vi "WPI_CameraGet Numeric Sensor Property.vi"(8 "error in (no error)":errorcluster, 10 "Property Name":string, 11 "CameraDevRef":T1) -> (0 "error out":errorcluster, 2 "Value":i32, 3 "CameraDevRef dup":T1)   [LabVIEW 2017]
doc: "This software is licensed. Open the labview\\readme\\WPI Robotics Library Open Source License.txt file for more information."
uses:
  <vilib>/Rock Robotics/WPI/Camera/WPI_CameraDevRef.ctl
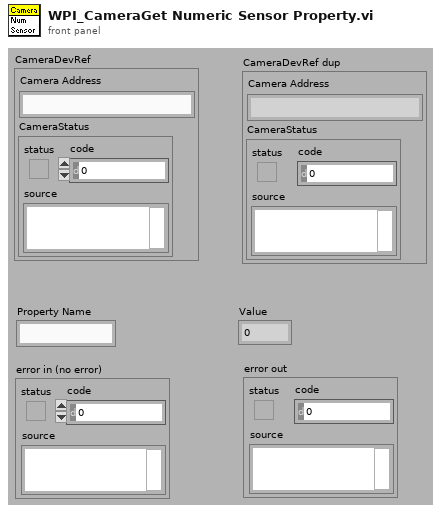
[diagram p1: front panel]
types:
  T1 = typedef "WPI_CameraDevRef.ctl" = cluster{"Camera Address":string, "CameraStatus":errorcluster}
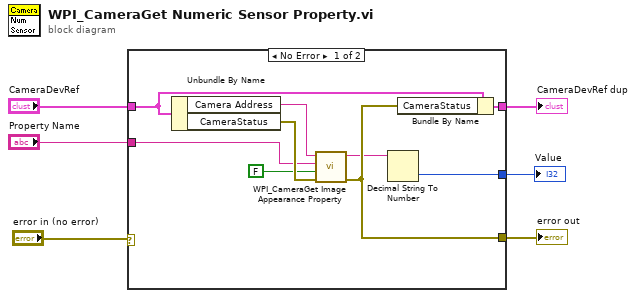
[diagram p0: block diagram]
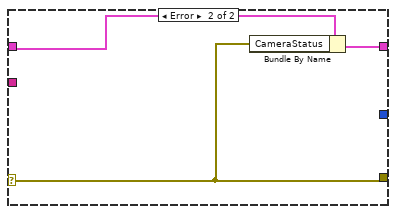
[diagram p2: hidden frame]
diagram:
  n1 = case shown="No Error" "error in (no error)" {
    selector: "error in (no error)" -> [_ w16]
    tunnel: "Property Name" -> [w10 _]
    tunnel: [w15 _] -> w5
    tunnel: [w11 w16] -> w4
    tunnel: "CameraDevRef" -> [w14 w17]
    tunnel: [w13 w18] -> w2
    frame No Error {
      n2 = Unbundle By Name(w14) -> ("Camera Address"=w9:string, "CameraStatus"=w12:errorcluster)
      n3 = call <vilib>:"WPI_CameraGet Image Appearance Property.vi"("error in (no error)"=w12, "Appearance"=FALSE, "Prop String"=w10, "address"=w9) -> ("error out"=w11:errorcluster, "Value"=w8:string)  [unwired: 6 in]
      n4 = Decimal String To Number(string=w8) -> (number=w15:i32)  [unwired: 3 out]
      n5 = Bundle By Name(cluster=w14, "CameraStatus"=w11) -> (w13:T1)
    }
    frame Error {
      n6 = Bundle By Name(cluster=w17, "CameraStatus"=w16) -> (w18:T1)
    }
  }
  "error out" <- w4
  "Value" <- w5
  "CameraDevRef dup" <- w2
